vi "GetN2.vi"(8 "error in (no error)":errorcluster, 11 "object in":refnum<class "Object (subject).lvclass">) -> (0 "error out":errorcluster, 2 "property":dbl, 3 "object out":refnum<class "Object (subject).lvclass">)   [LabVIEW 2014, in "Object (subject).lvclass"]
uses:
  Object (subject).lvclass
  Object (subject).lvclass/Object (subject).ctl
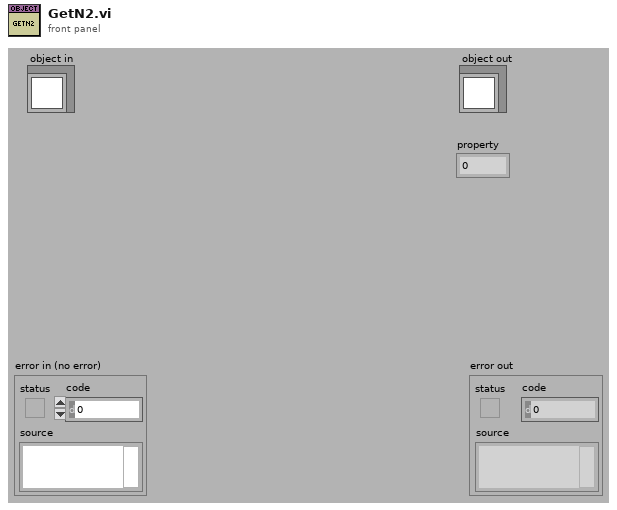
[diagram p1: front panel]
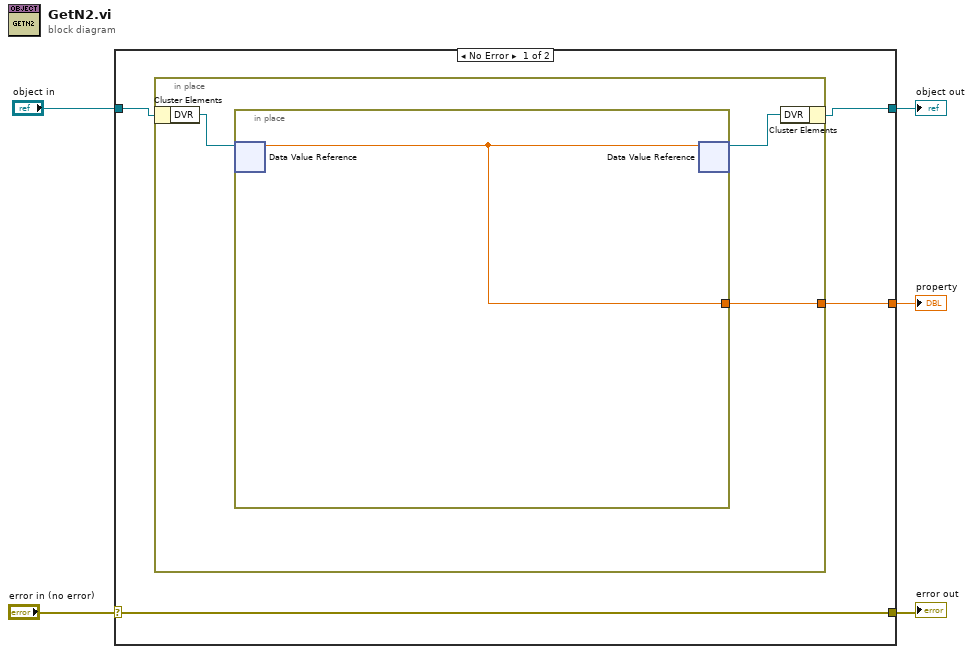
[diagram p0: block diagram]
diagram:
  n1 = case shown="No Error" "error in (no error)" {
    selector: "error in (no error)" -> [w8 w15]
    tunnel: [w8 w15] -> w4
    tunnel: [w6 w14] -> w2
    tunnel: "object in" -> [w7 w14]
    tunnel: [w9 _] -> w1
    frame No Error {
      n2 = in-place {
        in-place-border: [w10] -> w9
        n3 = in-place-cluster #1(w7) -> ("DVR"=w12:refnum<data-value>)
        n4 = in-place {
          in-place-border: [w13] -> w10
          n5 = in-place-dvr #2(w12) -> (w13:dbl)  [unwired: 1 out]
          n6 = in-place-dvr #2(w13) -> (w11:refnum<data-value>)  [unwired: 1 out]
        }
        n7 = in-place-cluster #1("DVR"=w11) -> (w6:refnum<class "Object (subject).lvclass">)
      }
    }
    frame Error {
    }
  }
  "error out" <- w4
  "object out" <- w2
  "property" <- w1
